vi "NextToken.vi"(8 "error in (no error)":errorcluster, 10 "Index In":i32, 11 "JSON String":string) -> (0 "error out":errorcluster, 1 "TOKEN":T1, 2 "Index Out":i32, 3 "JSON String Passthrough":string)   [LabVIEW 2017, in "Advanced Variant Tools.lvlib" / "JSON Support.lvlib"]
uses:
  JSON Support.lvlib
  Token Type.ctl
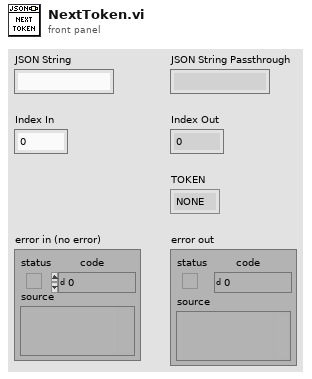
[diagram p1: front panel]
types:
  T1 = typedef "Advanced Variant Tools.lvlib/JSON Support.lvlib/Token Type.ctl" = enum16{"NONE", "CURLY_OPEN", "CURLY_CLOSE", "SQUARED_OPEN", "SQUARED_CLOSE", "COLON", "COMMA", "STRING", "NUMBER", "TRUE", "FALSE", "NULL"}
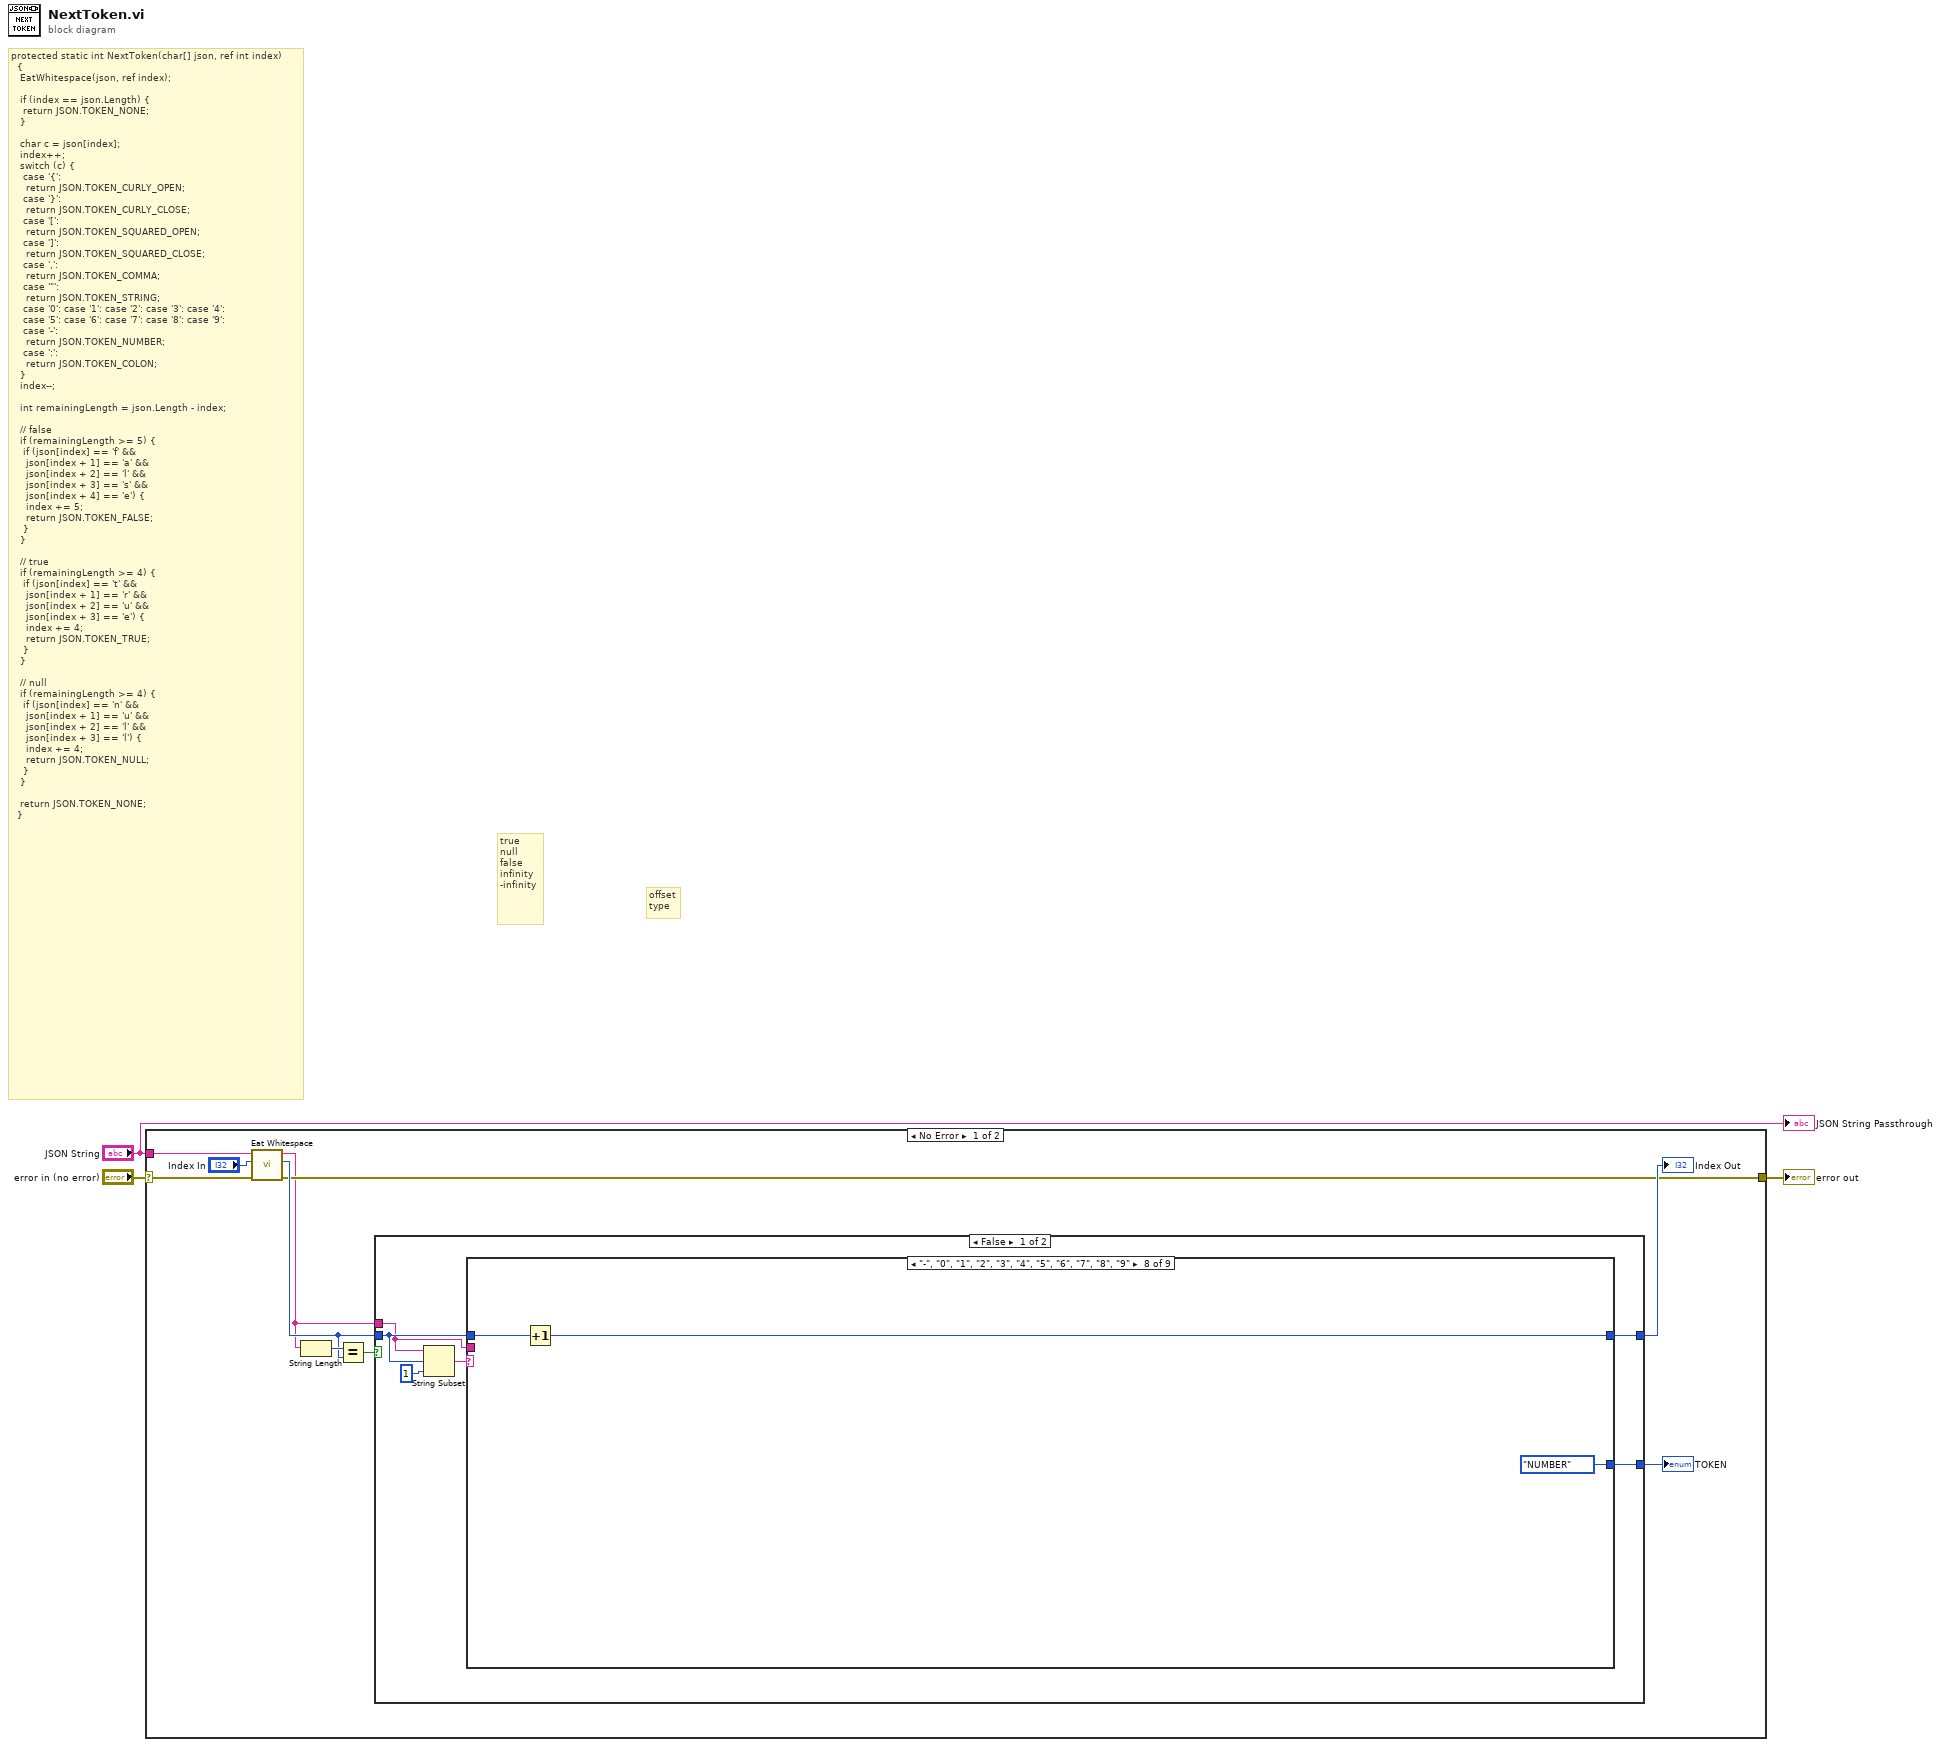
[diagram p0: block diagram]
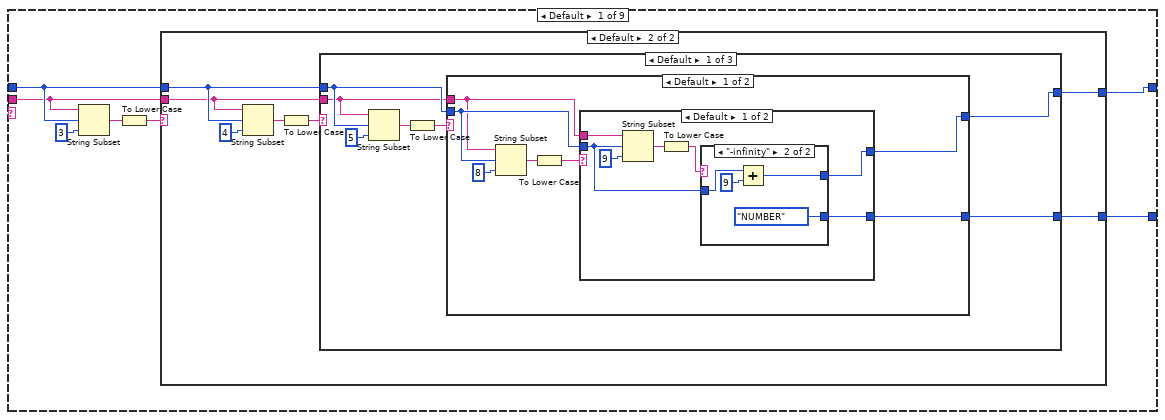
[diagram p2: hidden frame]
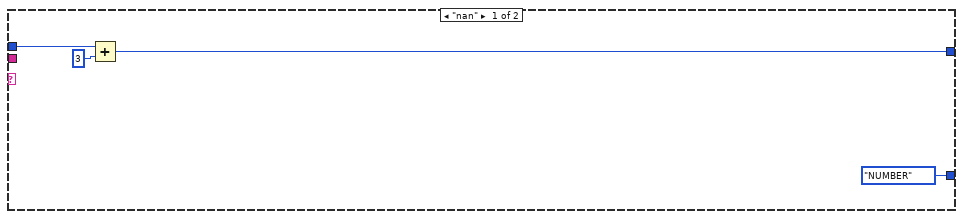
[diagram p3: hidden frame]
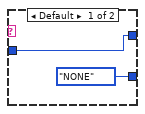
[diagram p4: hidden frame]
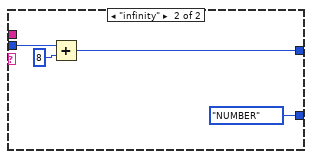
[diagram p5: hidden frame]
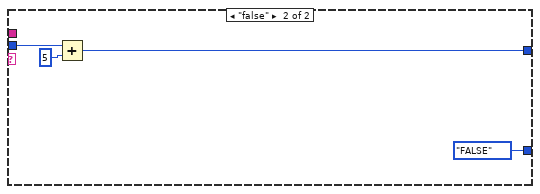
[diagram p6: hidden frame]
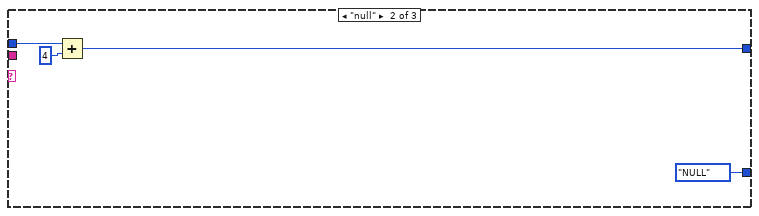
[diagram p7: hidden frame]
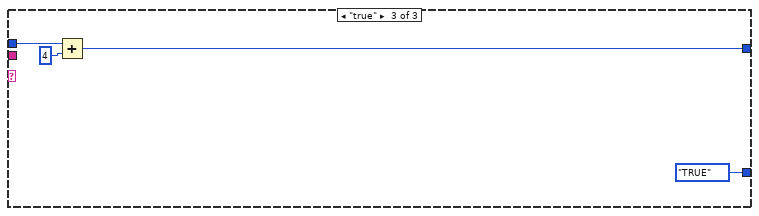
[diagram p8: hidden frame]
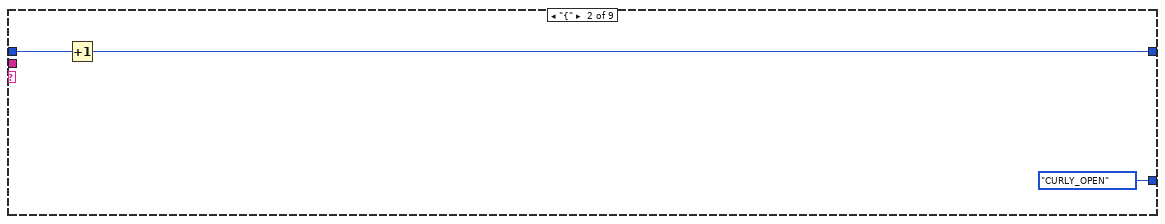
[diagram p9: hidden frame]
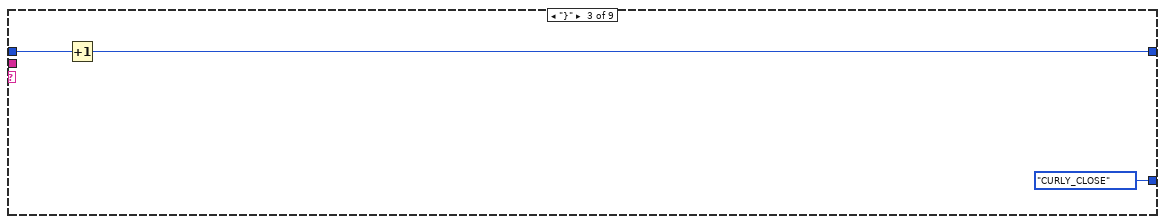
[diagram p10: hidden frame]
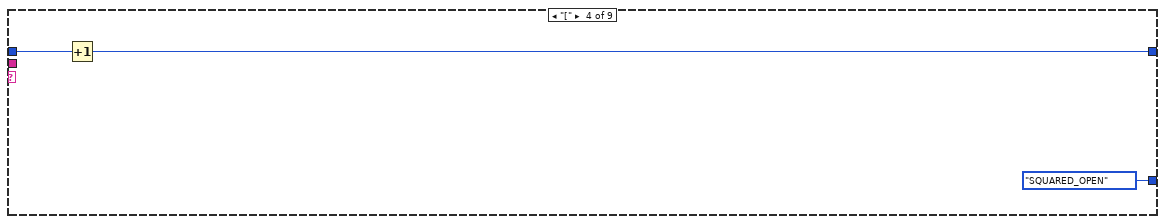
[diagram p11: hidden frame]
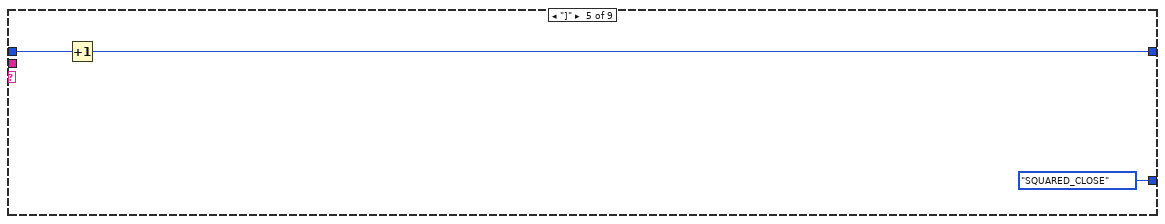
[diagram p12: hidden frame]
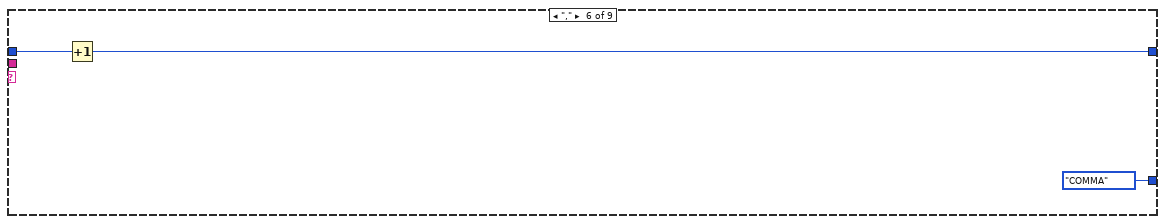
[diagram p13: hidden frame]
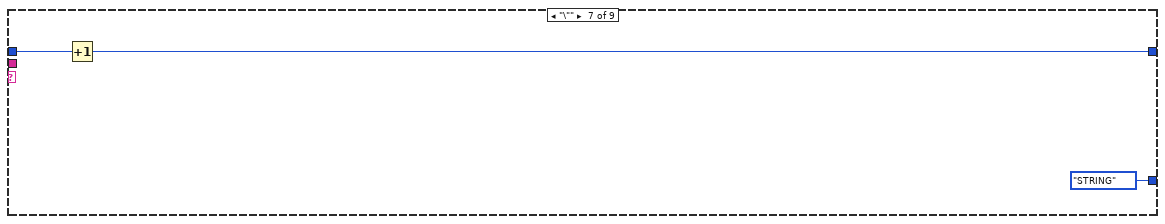
[diagram p14: hidden frame]
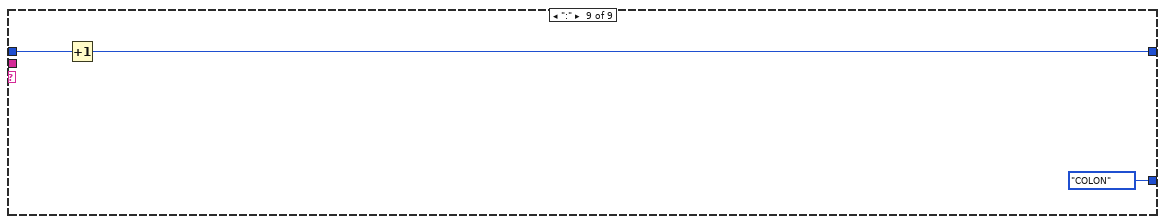
[diagram p15: hidden frame]
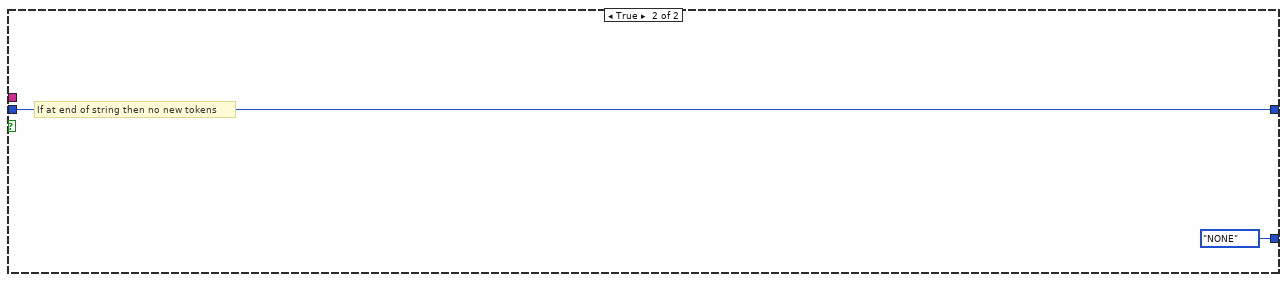
[diagram p16: hidden frame]
diagram:
  # "offset\ntype"
  # "true\nnull\nfalse\ninfinity\n-infinity"
  # "protected static int NextToken(char[] json, ref int index)\n\t\t{\n\t\t\tEatWhitespace(json, ref index);\n\n\t\t\tif (index == json.Length) {\n\t\t\t\treturn JSON.TOKEN_NONE;\n\t\t\t}\n\n\t\t\tchar c = json[index];\n\t\t\tindex++;\n\t\t\tswitch (c) {\n\t\t\t\tcase '{':\n\t\t\t\t\treturn JSON.TOKEN_CURLY_OPEN;\n\t\t\t\tcase '}':\n\t\t\t\t\treturn JSON.TOKEN_CURLY_CLOSE;\n\t\t\t\tcase '[':\n\t\t\t\t\treturn JSON.TOKEN_SQUARED_OPEN;\n\t\t\t\tcase ']':\n\t\t\t\t\treturn JSON.TOKEN_SQUARED_CLOSE;\n\t\t\t\tcase ',':\n\t\t\t\t\treturn JSON.TOKEN_COMMA;\n\t\t\t\tcase '\"':\n\t\t\t\t\treturn JSON.TOKEN_STRING;\n\t\t\t\tcase '0': case '1': case '2': case '3': case '4':\n\t\t\t\tcase '5': case '6': case '7': case '8': case '9':\n\t\t\t\tcase '-':\n\t\t\t\t\treturn JSON.TOKEN_NUMBER;\n\t\t\t\tcase ':':\n\t\t\t\t\treturn JSON.TOKEN_COLON;\n\t\t\t}\n\t\t\tindex--;\n\n\t\t\tint remainingLength = json.Length - index;\n\n\t\t\t// false\n\t\t\tif (remainingLength >= 5) {\n\t\t\t\tif (json[index] == 'f' &&\n\t\t\t\t\tjson[index + 1] == 'a' &&\n\t\t\t\t\tjson[index + 2] == 'l' &&\n\t\t\t\t\tjson[index + 3] == 's' &&\n\t\t\t\t\tjson[index + 4] == 'e') {\n\t\t\t\t\tindex += 5;\n\t\t\t\t\treturn JSON.TOKEN_FALSE;\n\t\t\t\t}\n\t\t\t}\n\n\t\t\t// true\n\t\t\tif (remainingLength >= 4) {\n\t\t\t\tif (json[index] == 't' &&\n\t\t\t\t\tjson[index + 1] == 'r' &&\n\t\t\t\t\tjson[index + 2] == 'u' &&\n\t\t\t\t\tjson[index + 3] == 'e') {\n\t\t\t\t\tindex += 4;\n\t\t\t\t\treturn JSON.TOKEN_TRUE;\n\t\t\t\t}\n\t\t\t}\n\n\t\t\t// null\n\t\t\tif (remainingLength >= 4) {\n\t\t\t\tif (json[index] == 'n' &&\n\t\t\t\t\tjson[index + 1] == 'u' &&\n\t\t\t\t\tjson[index + 2] == 'l' &&\n\t\t\t\t\tjson[index + 3] == 'l') {\n\t\t\t\t\tindex += 4;\n\t\t\t\t\treturn JSON.TOKEN_NULL;\n\t\t\t\t}\n\t\t\t}\n\n\t\t\treturn JSON.TOKEN_NONE;\n\t\t}"
  n1 = case shown="No Error" "error in (no error)" {
    selector: "error in (no error)" -> [w12 w107]
    tunnel: [w5 w107] -> w2
    tunnel: "JSON String" -> [w8 _]
    frame No Error {
      n2 = call "Eat Whitespace.vi"("error in (no error)"=w12, "Index In"="Index In", "JSON String"=w8) -> ("error out"=w5:errorcluster, "Index Out"=w7:i32, "JSON String Passthrough"=w4:string)  [unwired: 6 in]
      n3 = String Length(string=w4) -> (length=w11:i32)
      n4 = Equal?(x=w11, y=w7) -> (x = y?=w10:bool)
      n5 = case shown="False" w10 {
        tunnel: [w15 Token_Type."NONE" ("TOKEN")] -> w9
        tunnel: w7 -> [w17 w105]
        tunnel: w4 -> [w14 _]
        tunnel: [w16 w105] -> w6
        frame False {
          n6 = String Subset(string=w14, offset (0)=w17, length (rest)=1 ("length (rest)")) -> (substring=w18:string)
          n7 = case shown="\"-\", \"0\", \"1\", \"2\", \"3\", \"4\", \"5\", \"6\", \"7\", \"8\", \"9\"" w18 {
            tunnel: w17 -> [w23 w83 w85 w88 w90 w94 w97 w100 w103]
            tunnel: [w22 w82 w84 w87 w91 w93 w96 w99 w102] -> w16
            tunnel: [w21 Token_Type."CURLY_OPEN" ("TOKEN") Token_Type."CURLY_CLOSE" ("TOKEN") Token_Type."SQUARED_OPEN" ("TOKEN") Token_Type."SQUARED_CLOSE" ("TOKEN") Token_Type."COMMA" ("TOKEN") Token_Type."STRING" ("TOKEN") Token_Type."NUMBER" ("TOKEN") Token_Type."COLON" ("TOKEN")] -> w15
            tunnel: w14 -> [w20 _ _ _ _ _ _ _ _]
            frame Default {
              n8 = String Subset(string=w20, offset (0)=w23, length (rest)=3 ("length (rest)")) -> (substring=w25:string)
              n9 = To Lower Case(string=w25) -> (all lower case string=w24:string)
              n10 = case shown="Default" w24 {
                tunnel: w23 -> [w30 w34]
                tunnel: [w29 w33] -> w22
                tunnel: [Token_Type."NUMBER" ("TOKEN") w32] -> w21
                tunnel: w20 -> [_ w31]
                frame "nan" {
                  n11 = Add(x=w30, y=3) -> (x+y=w29:i32)
                }
                frame Default {
                  n12 = String Subset(string=w31, offset (0)=w34, length (rest)=4 ("length (rest)")) -> (substring=w37:string)
                  n13 = To Lower Case(string=w37) -> (all lower case string=w35:string)
                  n14 = case shown="Default" w35 {
                    tunnel: w34 -> [w39 w76 w80]
                    tunnel: [w40 w74 w78] -> w33
                    tunnel: [w41 Token_Type."NULL" ("TOKEN") Token_Type."TRUE" ("TOKEN")] -> w32
                    tunnel: w31 -> [w38 _ _]
                    frame Default {
                      n15 = String Subset(string=w38, offset (0)=w39, length (rest)=5 ("length (rest)")) -> (substring=w43:string)
                      n16 = To Lower Case(string=w43) -> (all lower case string=w42:string)
                      n17 = case shown="Default" w42 {
                        tunnel: w39 -> [w48 w72]
                        tunnel: [w46 w70] -> w40
                        tunnel: [w47 Token_Type."FALSE" ("TOKEN")] -> w41
                        tunnel: w38 -> [w45 _]
                        frame Default {
                          n18 = String Subset(string=w45, offset (0)=w48, length (rest)=8 ("length (rest)")) -> (substring=w50:string)
                          n19 = To Lower Case(string=w50) -> (all lower case string=w51:string)
                          n20 = case shown="Default" w51 {
                            tunnel: w48 -> [w54 w68]
                            tunnel: [w53 w66] -> w46
                            tunnel: [w52 Token_Type."NUMBER" ("TOKEN")] -> w47
                            tunnel: w45 -> [w55 _]
                            frame Default {
                              n21 = String Subset(string=w55, offset (0)=w54, length (rest)=9 ("length (rest)")) -> (substring=w57:string)
                              n22 = To Lower Case(string=w57) -> (all lower case string=w58:string)
                              n23 = case shown="\"-infinity\"" w58 {
                                tunnel: w54 -> [w59 w64]
                                tunnel: [w59 w62] -> w53
                                tunnel: [Token_Type."NONE" ("TOKEN") Token_Type."NUMBER" ("TOKEN")] -> w52
                                frame Default {
                                }
                                frame "-infinity" {
                                n24 = Add(x=w64, y=9) -> (x+y=w62:i32)
                                }
                              }
                            }
                            frame "infinity" {
                              n25 = Add(x=w68, y=8) -> (x+y=w66:i32)
                            }
                          }
                        }
                        frame "false" {
                          n26 = Add(x=w72, y=5) -> (x+y=w70:i32)
                        }
                      }
                    }
                    frame "null" {
                      n27 = Add(x=w76, y=4) -> (x+y=w74:i32)
                    }
                    frame "true" {
                      n28 = Add(x=w80, y=4) -> (x+y=w78:i32)
                    }
                  }
                }
              }
            }
            frame "{" {
              n29 = Increment(x=w83) -> (x+1=w82:i32)
            }
            frame "}" {
              n30 = Increment(x=w85) -> (x+1=w84:i32)
            }
            frame "[" {
              n31 = Increment(x=w88) -> (x+1=w87:i32)
            }
            frame "]" {
              n32 = Increment(x=w90) -> (x+1=w91:i32)
            }
            frame "," {
              n33 = Increment(x=w94) -> (x+1=w93:i32)
            }
            frame "\"" {
              n34 = Increment(x=w97) -> (x+1=w96:i32)
            }
            frame "-", "0", "1", "2", "3", "4", "5", "6", "7", "8", "9" {
              n35 = Increment(x=w100) -> (x+1=w99:i32)
            }
            frame ":" {
              n36 = Increment(x=w103) -> (x+1=w102:i32)
            }
          }
        }
        frame True {
          # "If at end of string then no new tokens"
        }
      }
      "Index Out" <- w6
      "TOKEN" <- w9
    }
    frame Error {
    }
  }
  "error out" <- w2
  "JSON String Passthrough" <- "JSON String"
